vi "Configure Valve Mode.vi"(8 "error in (no error)":errorcluster, 10 "valve mode":u8(ring) items=["normal", "closed", "purge"], 11 "MKS MF1 in":refnum<class "PL MKS MF1 USB.lvclass">) -> (0 "error out":errorcluster, 3 "MKS MF1 out":refnum<class "PL MKS MF1 USB.lvclass">)   [LabVIEW 2015, in "PL MKS MF1 USB.lvclass"]
doc: "Configures valve mode."
uses:
  PL MKS MF1 USB.lvclass
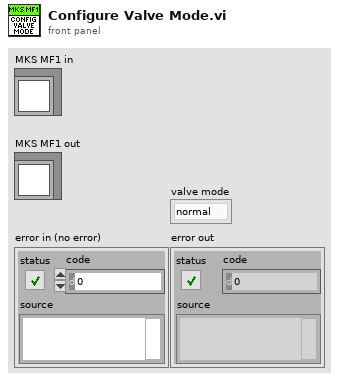
[diagram p1: front panel]
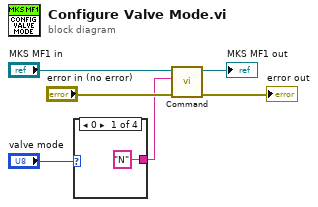
[diagram p0: block diagram]
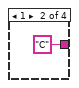
[diagram p2: hidden frame]
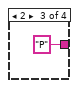
[diagram p3: hidden frame]
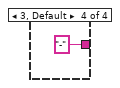
[diagram p4: hidden frame]
diagram:
  n1 = case shown="0" "valve mode" {
    tunnel: ["N" "C" "P" "-"] -> w1
    frame 0 {
    }
    frame 1 {
    }
    frame 2 {
    }
    frame 3, Default {
    }
  }
  n2 = call "Command.vi"("error in (no error)"="error in (no error)", "command"=w1, "MKS MF1 in"="MKS MF1 in") -> ("error out"=→"error out":errorcluster, "MKS MF1 out"=→"MKS MF1 out":refnum<class "PL MKS MF1 USB.lvclass">)  [unwired: 5 in, 2 out]
